vi "AI.Coupling.enum.convert.vi"(1 "AI.Coupling":enum16{"AC", "DC", "GND"}(ring)) -> (0 "Numeric":i32)   [LabVIEW 2016]
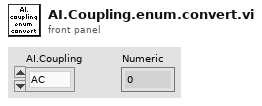
[diagram p1: front panel]
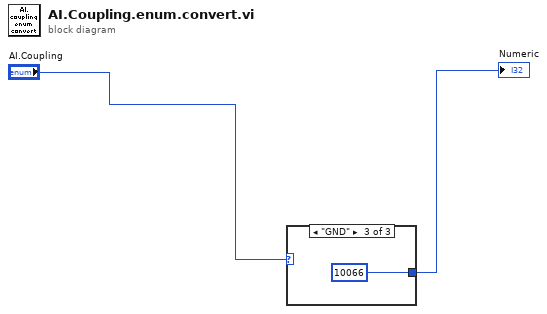
[diagram p0: block diagram]
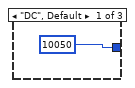
[diagram p2: hidden frame]
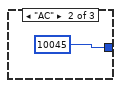
[diagram p3: hidden frame]
diagram:
  n1 = case shown="\"GND\"" "AI.Coupling" {
    tunnel: [10050 10045 10066] -> w2
    frame "DC", Default {
    }
    frame "AC" {
    }
    frame "GND" {
    }
  }
  "Numeric" <- w2
